vi "publisher tests Writer.vi"() -> ()   [LabVIEW 2018]
uses:
  publisher action.ctl
  publisher message.ctl
panel:
  out "Numeric":i32
  out "number":dbl
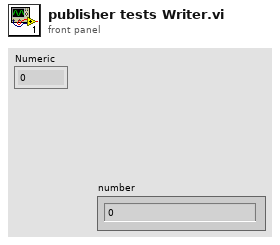
[diagram p1: front panel]
types:
  T1 = typedef "publisher action.ctl" = enum16{"set", "get", "init", "--send request", "--wait", "--respond", "init writer", "init reader"}
  T2 = typedef "publisher message.ctl" = cluster{"action":enum16{"next?", "ok"}, "data":dbl}
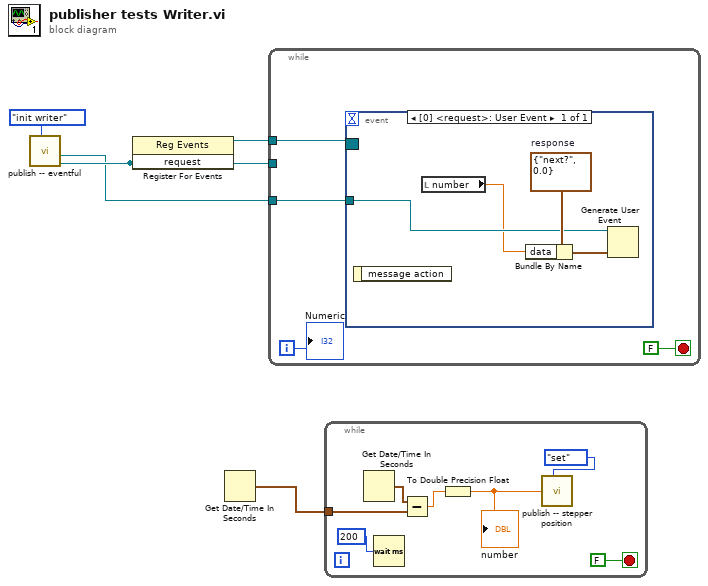
[diagram p0: block diagram]
diagram:
  n1 = call "publish -- eventful.vi"("publisher action"=publisher_action."init writer") -> ("request"=w4:refnum<user-event>, "response"=w3:refnum<user-event>)  [unwired: 8 in, 1 out]
  n2 = register-events(w4) -> (reference out=w5:refnum<event-registration>)  [unwired: 2 in, 1 out]
  n3 = Get Date/Time In Seconds() -> (seconds since 1Jan1904=w1:timestamp)
  n4 = while {
    tunnel: w5 -> [w7]
    tunnel: w4 -> [_]
    tunnel: w3 -> [w6]
    i -> [w8]
    stop <- FALSE stop-if-true
    n5 = event shown="[0] <request>: User Event" {
      selector: w7 -> [_]
      dyn-events: _ -> [_]
      timeout: _ -> [_]
      tunnel: w6 -> [w11]
      event User Event {
        w12 = T2 {"action"=enum."next?", "data"=0.0}  # response
        n6 = event-data() -> ()  [unwired: 1 in, 1 out]
        n7 = local read "number"() -> (w10:dbl)
        n8 = Bundle By Name(cluster=w12, "data"=w10) -> (w13:T2)
        n9 = Generate User Event(user event=w11, event data cluster=w13) -> ()  [unwired: 2 in, 2 out]
      }
    }
    "Numeric" <- w8
  }
  n10 = while {
    tunnel: w1 -> [w16]
    stop <- FALSE stop-if-true
    n11 = Get Date/Time In Seconds() -> (seconds since 1Jan1904=w19:timestamp)
    n12 = Wait (ms)(milliseconds to wait=u32 200) -> ()  [unwired: 1 out]
    n13 = Subtract(x=w19, y=w16) -> (x-y=w20:dbl)
    n14 = To Double Precision Float(number=w20) -> (double precision float=w18:dbl)
    "number" <- w18
    n15 = call "publish -- stepper position.vi"("publisher action"=publisher_action."set", "stepper pos IN"=w18) -> ()  [unwired: 9 in, 1 out]
  }
